vi "Instrument Status.vi"(8 "error in (no error)":errorcluster, 11 "VISA resource name":refnum<visa-resource-name>) -> (0 "error out":errorcluster, 1 "Key Status":u16, 2 "Lock Code":u16=123, 3 "VISA resource name out":refnum<visa-resource-name>, 4 "Remote Interface Mode":u16(ring) items=["Local", "Remote", "Remote with local lockout"], 5 "Keypad Locked":bool)   [LabVIEW 2019, in "Lake Shore 325.lvlib"]
doc: "This VI returns various instrument settings. Parameters returned are;\nRemote interface mode, key status, and keypad lock out."
uses:
  Lake Shore 325.lvlib
  Instance           1 25Saved   Instrument Status .vi
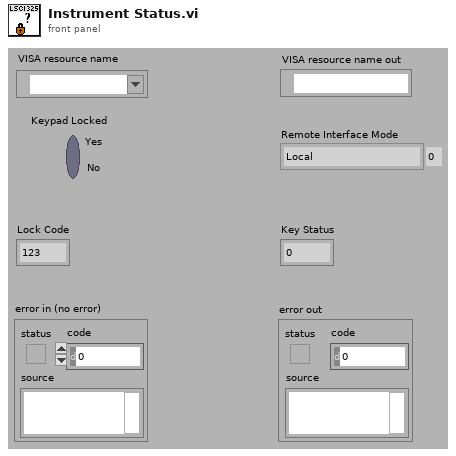
[diagram p1: front panel]
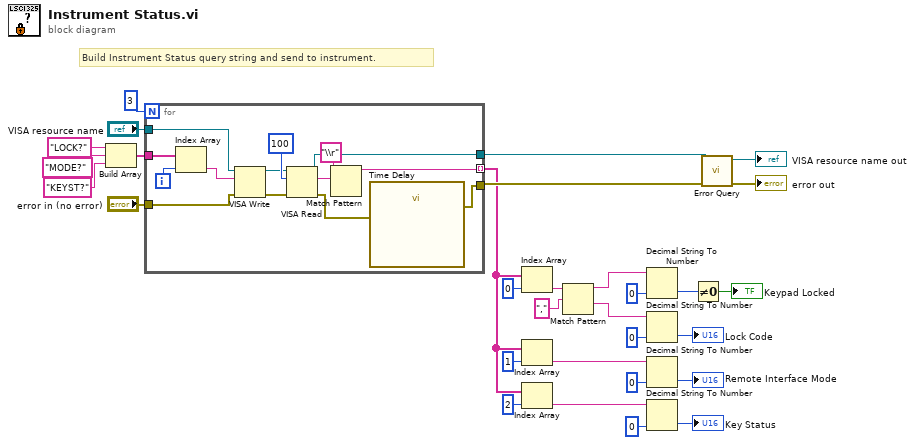
[diagram p0: block diagram]
diagram:
  # "Build Instrument Status query string and send to instrument."
  n1 = Build Array("LOCK?", "MODE?", "KEYST?") -> (w26:string[])
  n2 = for {
    N: 3 -> [_]
    tunnel: [w38] -> w25
    tunnel: [w32] -> w24
    tunnel: "VISA resource name" -> [w37]
    tunnel: "error in (no error)" -> [w36]
    tunnel: w26 -> [w35]
    tunnel: [w34] -> w16 mode=indexing
    i -> [w39]
    n3 = Index Array(array=w35, index=w39) -> (element=w33:string)
    n4 = VISA Write(VISA resource name=w37, write buffer=w33, error in (no error)=w36) -> (VISA resource name out=w41:refnum<visa-resource-name>, error out=w40:errorcluster)  [unwired: 1 out]
    n5 = VISA Read(VISA resource name=w41, byte count=100, error in (no error)=w40) -> (VISA resource name out=w38:refnum<visa-resource-name>, read buffer=w43:string, error out=w31:errorcluster)  [unwired: 1 out]
    n6 = Match Pattern(string=w43, regular expression="\\r") -> (before substring=w34:string)  [unwired: 1 in, 3 out]
    n7 = call "Time Delay"("error in (no error)"=w31) -> ("error out"=w32:errorcluster)  [unwired: 10 in]
  }
  n8 = Index Array(array=w16, index=0) -> (element=w18:string)
  n9 = Index Array(array=w16, index=1) -> (element=w14:string)
  n10 = Index Array(array=w16, index=2) -> (element=w12:string)
  n11 = Match Pattern(string=w18, regular expression=",") -> (before substring=w6:string, after substring=w4:string)  [unwired: 1 in, 2 out]
  n12 = Decimal String To Number(string=w6, default (0L)=u16 0) -> (number=w7:u16)  [unwired: 1 in, 1 out]
  n13 = Decimal String To Number(string=w4, default (0L)=u16 0) -> (number=→"Lock Code":u16)  [unwired: 1 in, 1 out]
  n14 = Decimal String To Number(string=w14, default (0L)=u16 0) -> (number=→"Remote Interface Mode":u16)  [unwired: 1 in, 1 out]
  n15 = Decimal String To Number(string=w12, default (0L)=0) -> (number=→"Key Status":i32)  [unwired: 1 in, 1 out]
  n16 = Not Equal To 0?(x=w7) -> (x != 0?=→"Keypad Locked":bool)
  n17 = call "Error Query.vi"("error in (no error)"=w24, "VISA resource name"=w25) -> ("error out"=→"error out":errorcluster, "VISA resource name out"=→"VISA resource name out":refnum<visa-resource-name>)  [unwired: 7 in, 1 out]
